vi "DEMO.vi"() -> ()   [LabVIEW 2012, in "Array Stack.lvlib"]
uses:
  Array Stack.lvlib
panel:
  out "出栈":dbl[](array[numeric])
  out "因数":dbl[](array[numeric])
  in  "数值":i32
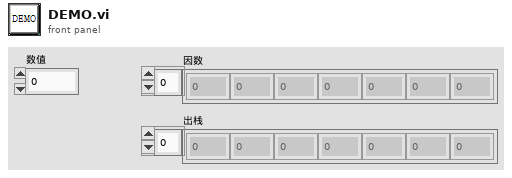
[diagram p1: front panel]
types:
  T1 = typedef "Array Stack.lvlib/堆栈操作.ctl" = enum16{"初始化（Init）", "进栈（Push）", "出栈（Pop）", "状态（Status)", "释放"}
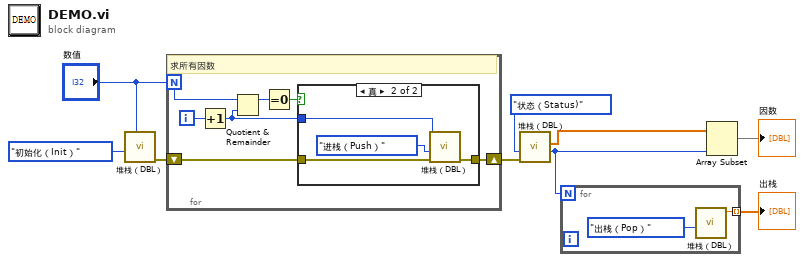
[diagram p0: block diagram]
diagram:
  n1 = call "堆栈（DBL）.vi"("堆栈长度"="数值", "堆栈操作"=堆栈操作."初始化（Init）") -> ("error out"=w7:errorcluster)  [unwired: 4 in, 5 out]
  n2 = for {
    N: "数值" -> [w15]
    shift-right: [w10] -> w6
    shift-left: w7 -> [w12]
    i -> [w16]
    # "求所有因数"
    n3 = Increment(x=w16) -> (x+1=w11:i32)
    n4 = Quotient & Remainder(x=w15, y=w11) -> (x-y*floor(x/y)=w14:i32)  [unwired: 1 out]
    n5 = Equal To 0?(x=w14) -> (x = 0?=w13:bool)
    n6 = case shown="真" w13 {
      tunnel: w12 -> [w17 w21]
      tunnel: w11 -> [_ w19]
      tunnel: [w17 w18] -> w10
      frame False {
      }
      frame True {
        n7 = call "堆栈（DBL）.vi"("error in (no error)"=w21, "堆栈操作"=堆栈操作."进栈（Push）", "入栈元素(DBL)"=w19) -> ("error out"=w18:errorcluster)  [unwired: 3 in, 5 out]
      }
    }
  }
  n8 = call "堆栈（DBL）.vi"("error in (no error)"=w6, "堆栈操作"=堆栈操作."状态（Status)") -> ("已用堆栈长度"=w2:i32, "预览"=w4:dbl[])  [unwired: 4 in, 4 out]
  n9 = for {
    N: w2 -> [_]
    tunnel: [w22] -> w1 mode=indexing
    n10 = call "堆栈（DBL）.vi"("堆栈操作"=堆栈操作."出栈（Pop）") -> ("出栈元素"=w22:dbl)  [unwired: 5 in, 5 out]
  }
  "出栈" <- w1
  n11 = Array Subset(array=w4, length=w2) -> (→"因数":dbl[])  [unwired: 1 in]
